vi "GetOuterTunnels.vi"(6 "error in":errorcluster, 9 "FlatSequenceFrame in":refnum<class "FlatSequenceFrame.lvclass">) -> (0 "error out":errorcluster, 3 "FlatSequenceFrame out":refnum<class "FlatSequenceFrame.lvclass">, 4 "outside tunnels":i32[](array[numeric]))   [LabVIEW 2014, in "FlatSequenceFrame.lvclass"]
uses:
  FlatSequenceFrame.lvclass
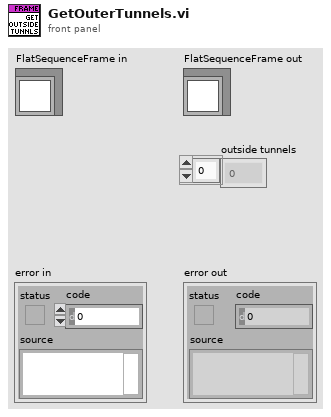
[diagram p1: front panel]
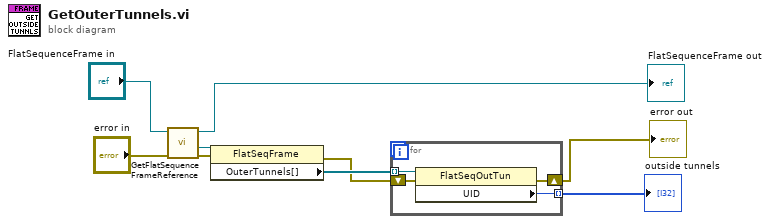
[diagram p0: block diagram]
diagram:
  n1 = call "GetFlatSequenceFrameReference.vi"("error in"="error in", "FlatSequence in"="FlatSequenceFrame in") -> ("error out"=w6:errorcluster, "reference out"=w7:refnum<vi>, "FlatSequence out"=→"FlatSequenceFrame out":refnum<class "FlatSequenceFrame.lvclass">)  [unwired: 7 in]
  n2 = property class="FlatSeqFrame"(reference=w7, error in=w6) -> (error out=w2:errorcluster, "OuterTunnels[]"=w4:refnum<vi>[])  [unwired: 1 out]
  n3 = for {
    tunnel: w4 -> [w13] mode=indexing
    shift-right: [w11] -> w1
    shift-left: w2 -> [w12]
    tunnel: [w10] -> w3 mode=indexing
    n4 = property class="FlatSeqOutTun"(reference=w13, error in=w12) -> (error out=w11:errorcluster, "UID"=w10:i32)  [unwired: 1 out]
  }
  "error out" <- w1
  "outside tunnels" <- w3
